vi "LVClass_SlopesPostProcessList AddProcessorTabWithVaraint.vi"(0 "SlopesPostProcessorList in":refnum<class "SlopesPostProcessorList.lvclass">, 7 "Processing list in":T1[](array[typedef]), 9 "Enum":enum16{"As new list", "Append", "InsertFront"}(ring), 11 "error in":errorcluster) -> (4 "SlopesPostProcessorList out":refnum<class "SlopesPostProcessorList.lvclass">, 15 "error out":errorcluster)   [LabVIEW 2020, in "SlopesPostProcessorList.lvclass"]
uses:
  SlopesPostProcessorList.lvclass
  SlopesPostProcessorList - ONE - with variant.ctl
  SlopesStructToVariant.ctl
  Point2D.ctl
  Point2Df.ctl
  Slopes origin - SlopesPostProcessingList.ctl
  HasoSlopes.lvclass
  PupillStructToVariant.ctl
  General dimensions definition.ctl
  Pupil.lvclass
  SlopesPostProcessorList - Double passage.ctl
  SlopesPostProcessorList - Filter.ctl
  SlopesPostProcessorList - Modulator.ctl
  SlopesPostProcessorList - Add lens.ctl
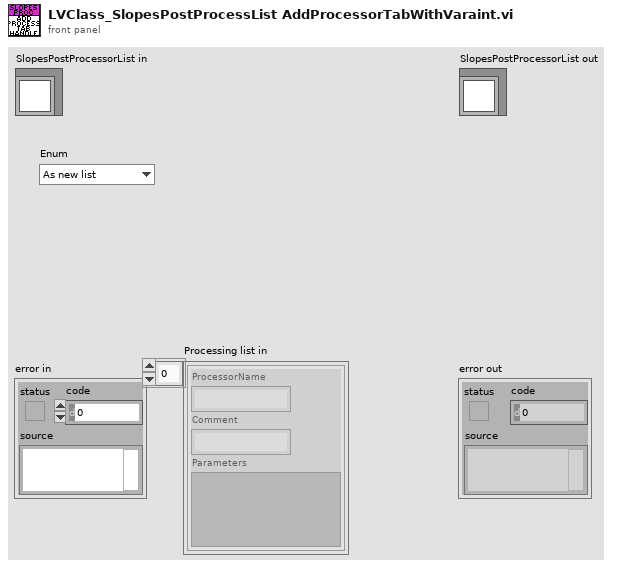
[diagram p1: front panel]
types:
  T1 = typedef "SlopesPostProcessorList - ONE - with variant.ctl" = cluster{"ProcessorName":string, "Comment":string, "Parameters":variant}
  T2 = typedef "SlopesPostProcessorList - Double passage.ctl" = cluster{"ActivateOnTilt":bool, "ActivateOnCurvature":bool}
  T3 = typedef "SlopesPostProcessorList - Filter.ctl" = cluster{"tiltx":bool, "tilty":bool, "curv":bool, "astig0":bool, "astig45":bool, "others":bool}
  T4 = typedef "SlopesPostProcessorList - Modulator.ctl" = cluster{"tiltx":sgl, "tilty":sgl, "curv":sgl, "astig0":sgl, "astig45":sgl, "others":sgl}
  T5 = typedef "SlopesPostProcessorList - Add lens.ctl" = cluster{"lens_m":sgl, "KeepCurvature":bool}
  T6 = typedef "SlopesStructToVariant.ctl" = cluster{"dimension":cluster{"size":T7, "step":T8}, "HASO serial number":string, "REF Type":T9, "Slopes from XML string format":string}
  T7 = typedef "Point2D.ctl" = cluster{"X":u32, "Y":u32}
  T8 = typedef "Point2Df.ctl" = cluster{"X":sgl, "Y":sgl}
  T9 = typedef "Slopes origin - SlopesPostProcessingList.ctl" = enum16{"Slopes from acq", "Slopes from file", "Slopes from data"}
  T10 = typedef "PupillStructToVariant.ctl" = cluster{"Dimension":T11, "Data":i32[][]}
  T11 = typedef "General dimensions definition.ctl" = cluster{"Size":T7, "Step":T8}
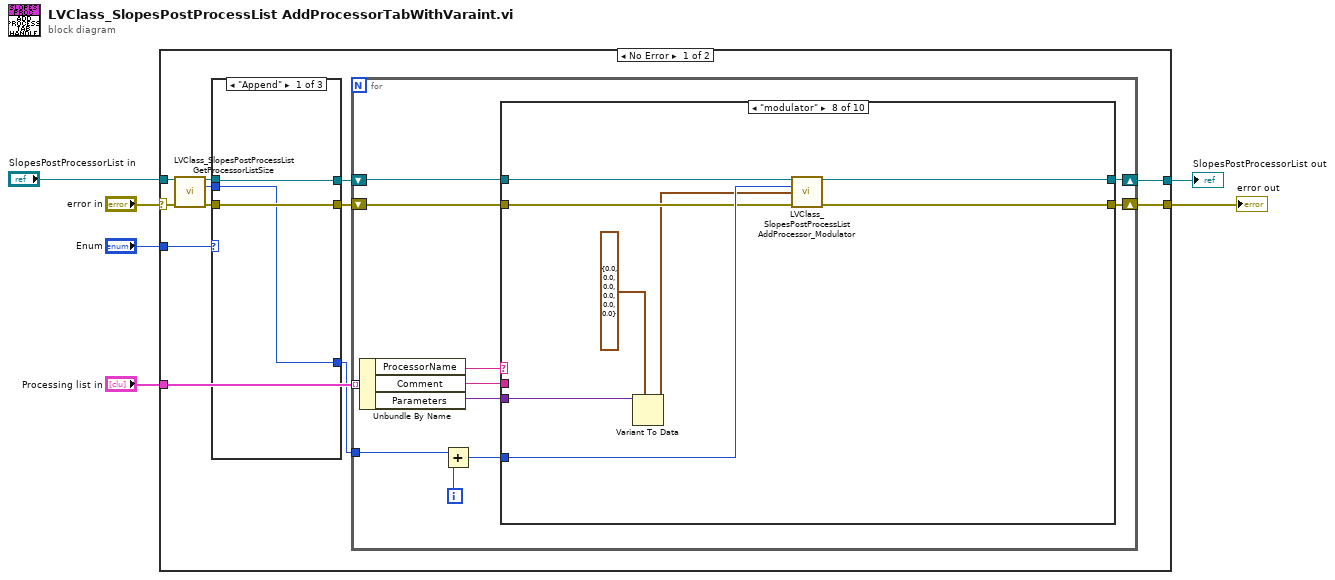
[diagram p0: block diagram]
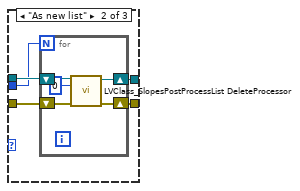
[diagram p2: hidden frame]
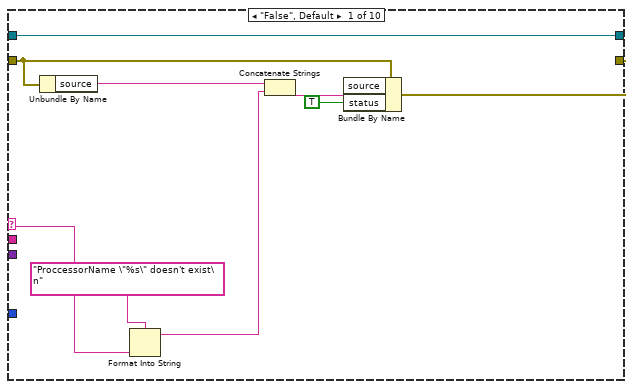
[diagram p4: hidden frame]
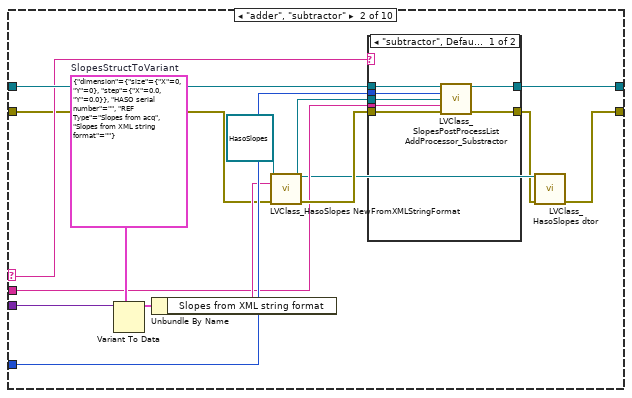
[diagram p5: hidden frame]
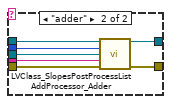
[diagram p6: hidden frame]
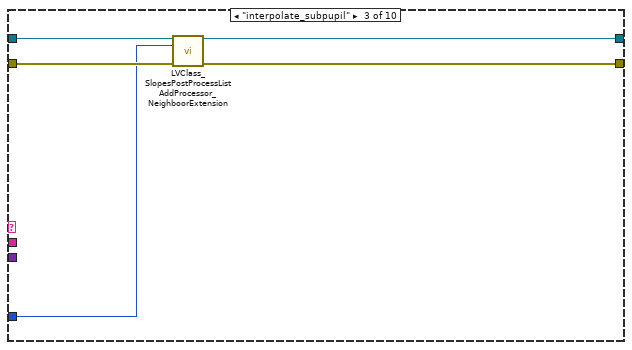
[diagram p7: hidden frame]
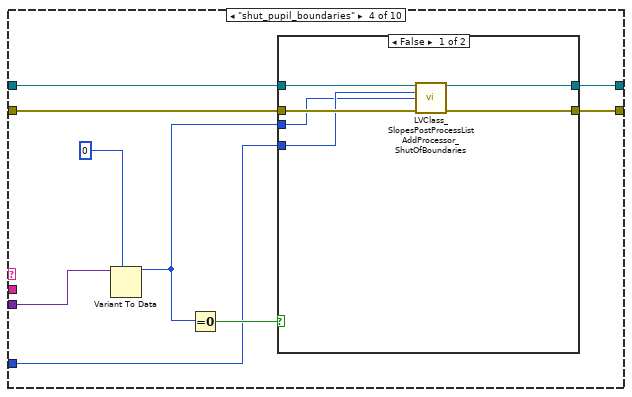
[diagram p8: hidden frame]
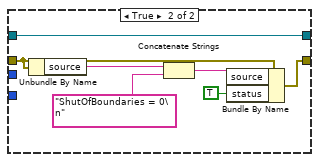
[diagram p9: hidden frame]
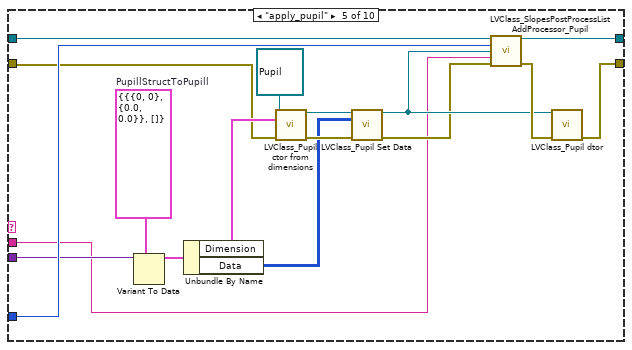
[diagram p10: hidden frame]
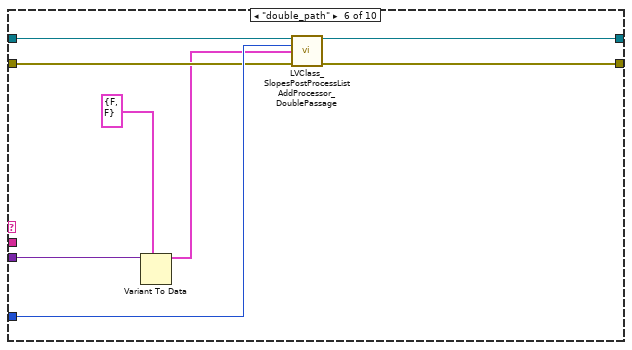
[diagram p11: hidden frame]
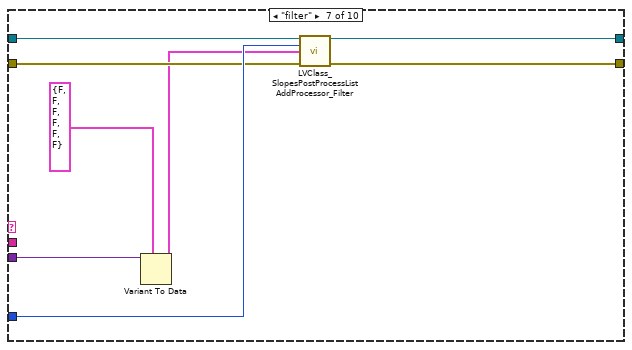
[diagram p12: hidden frame]
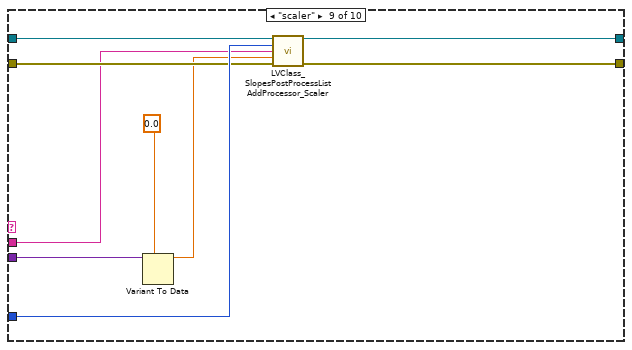
[diagram p13: hidden frame]
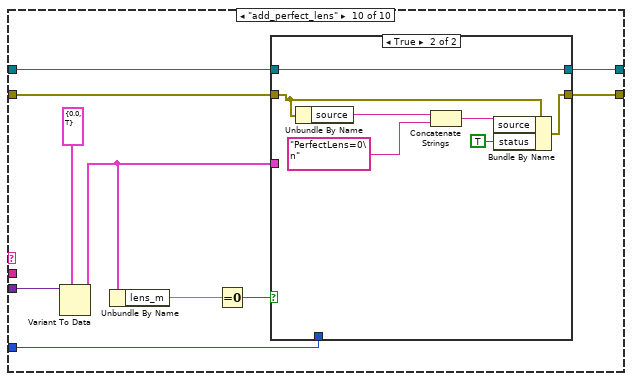
[diagram p14: hidden frame]
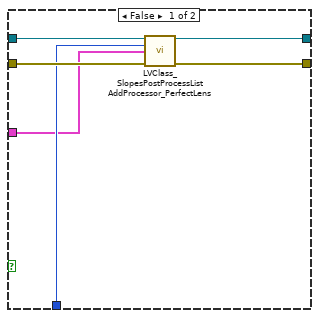
[diagram p15: hidden frame]
diagram:
  n1 = case shown="No Error" "error in" {
    selector: "error in" -> [w15 w184]
    tunnel: [w16 w184] -> w5
    tunnel: [w17 w183] -> w6
    tunnel: "SlopesPostProcessorList in" -> [w14 w183]
    tunnel: "Processing list in" -> [w18 _]
    tunnel: "Enum" -> [w9 _]
    frame No Error {
      n2 = call "LVClass_SlopesPostProcessList GetProcessorListSize.vi"("SlopesPostProcessorList in"=w14, "error in (no error)"=w15) -> ("SlopesPostProcessorList out"=w13:refnum<class "SlopesPostProcessorList.lvclass">, "size"=w8:u32, "error out"=w11:errorcluster)  [unwired: 11 in]
      n3 = case shown="\"Append\"" w9 {
        tunnel: w13 -> [w21 w26 w33]
        tunnel: [w21 w25 w33] -> w12
        tunnel: w11 -> [w20 w24 w32]
        tunnel: [w20 w23 w32] -> w10
        tunnel: w8 -> [w19 w22 _]
        tunnel: [w19 _ _] -> w7
        frame "Append" {
        }
        frame "As new list" {
          n4 = for {
            N: w22 -> [_]
            shift-right: [w30] -> w25
            shift-left: w26 -> [w31]
            shift-right: [w28] -> w23
            shift-left: w24 -> [w29]
            n5 = call "LVClass_SlopesPostProcessList DeleteProcessor.vi"("SlopesPostProcessorList in"=w31, "Position"=0, "error in (no error)"=w29) -> ("SlopesPostProcessorList out"=w30:refnum<class "SlopesPostProcessorList.lvclass">, "error out"=w28:errorcluster)  [unwired: 11 in]
          }
        }
        frame "InsertFront" {
        }
      }
      n6 = for {
        tunnel: w18 -> [w35] mode=indexing
        shift-right: [w42] -> w16
        shift-left: w10 -> [w43]
        shift-right: [w40] -> w17
        shift-left: w12 -> [w41]
        tunnel: w7 -> [w37]
        i -> [w39]
        n7 = Unbundle By Name(w35) -> ("ProcessorName"=w44:string, "Comment"=w34:string, "Parameters"=w36:variant)
        n8 = Add(x=w37, y=w39) -> (x+y=w38:u32)
        n9 = case shown="\"modulator\"" w44 {
          selector: w44 -> [w45 w65 _ _ _ _ _ _ _ _]
          tunnel: w43 -> [w53 w59 w85 w95 w113 w131 w139 w147 w156 w168]
          tunnel: [w52 w54 w84 w94 w120 w130 w137 w145 w155 w169] -> w42
          tunnel: w38 -> [_ w66 w83 w91 w125 w134 w141 w149 w157 w164]
          tunnel: w41 -> [w46 w68 w87 w93 w124 w133 w140 w148 w159 w166]
          tunnel: [w46 w67 w86 w92 w126 w132 w138 w146 w158 w165] -> w40
          tunnel: w36 -> [_ w63 _ w88 w122 w128 w142 w150 w152 w163]
          tunnel: w34 -> [_ w57 _ _ w110 _ _ _ w154 _]
          frame "False", Default {
            n10 = Unbundle By Name(w53) -> ("source"=w50:string)
            n11 = Format Into String(format string="ProccessorName \"%s\" doesn't exist\n" ("source"), w45) -> (resulting string=w48:string)  [unwired: 2 in, 1 out]
            n12 = Concatenate Strings(w50, w48) -> (w49:string)
            n13 = Bundle By Name(cluster=w53, "source"=w49, "status"=TRUE) -> (w52:errorcluster)
          }
          frame "adder", "subtractor" {
            w64 = T6 {"dimension"={"size"={"X"=0, "Y"=0}, "step"={"X"=0.0, "Y"=0.0}}, "HASO serial number"="", "REF Type"=enum."Slopes from acq", "Slopes from XML string format"=""}  # SlopesStructToVariant
            n14 = Variant To Data(type=w64, Variant=w63) -> (data=w62:T6)  [unwired: 1 in, 1 out]
            n15 = Unbundle By Name(w62) -> ("Slopes from XML string format"=w61:string)
            n16 = call "LVClass_HasoSlopes NewFromXMLStringFormat.vi"("HasoSlopes in"=refnum<class "HasoSlopes.lvclass"> refnum, "XML txt format"=w61, "error in (no error)"=w59) -> ("HasoSlopes out"=w56:refnum<class "HasoSlopes.lvclass">, "error out"=w58:errorcluster)  [unwired: 11 in]
            n17 = case shown="\"subtractor\", Default" w65 {
              tunnel: w68 -> [w75 w82]
              tunnel: [w70 w81] -> w67
              tunnel: w66 -> [w74 w80]
              tunnel: w57 -> [w72 w79]
              tunnel: w56 -> [w73 w78]
              tunnel: w58 -> [w71 w77]
              tunnel: [w69 w76] -> w55
              frame "subtractor", Default {
                n18 = call "LVClass_SlopesPostProcessList AddProcessor_Substractor.vi"("SlopesPostProcessorList in"=w75, "Position"=w74, "HasoSlopes.lvclass"=w73, "Comment"=w72, "error in (no error)"=w71) -> ("SlopesPostProcessorList out"=w70:refnum<class "SlopesPostProcessorList.lvclass">, "error out"=w69:errorcluster)  [unwired: 9 in]
              }
              frame "adder" {
                n19 = call "LVClass_SlopesPostProcessList AddProcessor_Adder.vi"("SlopesPostProcessorList in"=w82, "Position"=w80, "HasoSlopes.lvclass"=w78, "Comment"=w79, "error in (no error)"=w77) -> ("SlopesPostProcessorList out"=w81:refnum<class "SlopesPostProcessorList.lvclass">, "error out"=w76:errorcluster)  [unwired: 9 in]
              }
            }
            n20 = call "LVClass_HasoSlopes dtor.vi"("HasoSlopes in"=w56, "error in (no error)"=w55) -> ("error out"=w54:errorcluster)  [unwired: 12 in, 1 out]
          }
          frame "interpolate_subpupil" {
            n21 = call "LVClass_SlopesPostProcessList AddProcessor_NeighboorExtension.vi"("SlopesPostProcessorList in"=w87, "Position"=w83, "error in (no error)"=w85) -> ("SlopesPostProcessorList out"=w86:refnum<class "SlopesPostProcessorList.lvclass">, "error out"=w84:errorcluster)  [unwired: 11 in]
          }
          frame "shut_pupil_boundaries" {
            n22 = Variant To Data(type=u32 0 ("ShutOfBoundaries"), Variant=w88) -> (data=w89:u32)  [unwired: 1 in, 1 out]
            n23 = Equal To 0?(x=w89) -> (x = 0?=w96:bool)
            n24 = case shown="False" w96 {
              tunnel: w95 -> [w101 w104]
              tunnel: [w100 w105] -> w94
              tunnel: w93 -> [w102 w103]
              tunnel: [w99 w103] -> w92
              tunnel: w91 -> [w98 _]
              tunnel: w89 -> [w97 _]
              frame False {
                n25 = call "LVClass_SlopesPostProcessList AddProcessor_ShutOfBoundaries.vi"("SlopesPostProcessorList in"=w102, "Position"=w98, "ShutOfBoundaries"=w97, "error in (no error)"=w101) -> ("SlopesPostProcessorList out"=w99:refnum<class "SlopesPostProcessorList.lvclass">, "error out"=w100:errorcluster)  [unwired: 10 in]
              }
              frame True {
                n26 = Unbundle By Name(w104) -> ("source"=w108:string)
                n27 = Concatenate Strings(w108, "ShutOfBoundaries = 0\n" ("source")) -> (w107:string)
                n28 = Bundle By Name(cluster=w104, "source"=w107, "status"=TRUE) -> (w105:errorcluster)
              }
            }
          }
          frame "apply_pupil" {
            w123 = T10 {"Dimension"={"Size"={"X"=0, "Y"=0}, "Step"={"X"=0.0, "Y"=0.0}}, "Data"=[]}  # PupillStructToPupill
            n29 = Variant To Data(type=w123, Variant=w122) -> (data=w115:T10)  [unwired: 1 in, 1 out]
            n30 = Unbundle By Name(w115) -> ("Dimension"=w114:T11, "Data"=w111:i32[][])
            n31 = call "LVClass_Pupil ctor from dimensions.vi"("Pupil in"=refnum<class "Pupil.lvclass"> refnum, "Dimensions_um"=w114, "error in (no error)"=w113) -> ("Pupil out"=w116:refnum<class "Pupil.lvclass">, "error out"=w117:errorcluster)  [unwired: 11 in]
            n32 = call "LVClass_Pupil Set Data.vi"("Pupil in"=w116, "Data"=w111, "error in (no error)"=w117) -> ("Pupil out"=w119:refnum<class "Pupil.lvclass">, "error out"=w118:errorcluster)  [unwired: 11 in]
            n33 = call "LVClass_SlopesPostProcessList AddProcessor_Pupil.vi"("SlopesPostProcessorList in"=w124, "Position"=w125, "Pupil.lvclass"=w119, "Comment"=w110, "error in (no error)"=w118) -> ("SlopesPostProcessorList out"=w126:refnum<class "SlopesPostProcessorList.lvclass">, "error out"=w121:errorcluster)  [unwired: 9 in]
            n34 = call "LVClass_Pupil dtor.vi"("Pupil in"=w119, "error in (no error)"=w121) -> ("error out"=w120:errorcluster)  [unwired: 12 in, 1 out]
          }
          frame "double_path" {
            n35 = Variant To Data(type=T2 {"ActivateOnTilt"=FALSE, "ActivateOnCurvature"=FALSE} ("doublePassage"), Variant=w128) -> (data=w127:T2)  [unwired: 1 in, 1 out]
            n36 = call "LVClass_SlopesPostProcessList AddProcessor_DoublePassage.vi"("SlopesPostProcessorList in"=w133, "Position"=w134, "doublePath"=w127, "error in (no error)"=w131) -> ("SlopesPostProcessorList out"=w132:refnum<class "SlopesPostProcessorList.lvclass">, "error out"=w130:errorcluster)  [unwired: 10 in]
          }
          frame "filter" {
            n37 = Variant To Data(type=T3 {"tiltx"=FALSE, "tilty"=FALSE, "curv"=FALSE, "astig0"=FALSE, "astig45"=FALSE, "others"=FALSE} ("Filter"), Variant=w142) -> (data=w135:T3)  [unwired: 1 in, 1 out]
            n38 = call "LVClass_SlopesPostProcessList AddProcessor_Filter.vi"("SlopesPostProcessorList in"=w140, "Position"=w141, "Filter"=w135, "error in (no error)"=w139) -> ("SlopesPostProcessorList out"=w138:refnum<class "SlopesPostProcessorList.lvclass">, "error out"=w137:errorcluster)  [unwired: 10 in]
          }
          frame "modulator" {
            n39 = Variant To Data(type=T4 {"tiltx"=0.0, "tilty"=0.0, "curv"=0.0, "astig0"=0.0, "astig45"=0.0, "others"=0.0} ("Modulator"), Variant=w150) -> (data=w143:T4)  [unwired: 1 in, 1 out]
            n40 = call "LVClass_SlopesPostProcessList AddProcessor_Modulator.vi"("SlopesPostProcessorList in"=w148, "Position"=w149, "Modulator"=w143, "error in (no error)"=w147) -> ("SlopesPostProcessorList out"=w146:refnum<class "SlopesPostProcessorList.lvclass">, "error out"=w145:errorcluster)  [unwired: 10 in]
          }
          frame "scaler" {
            n41 = Variant To Data(type=sgl 0.0 ("scaler"), Variant=w152) -> (data=w151:sgl)  [unwired: 1 in, 1 out]
            n42 = call "LVClass_SlopesPostProcessList AddProcessor_Scaler.vi"("SlopesPostProcessorList in"=w159, "Position"=w157, "comment"=w154, "scaler"=w151, "error in (no error)"=w156) -> ("SlopesPostProcessorList out"=w158:refnum<class "SlopesPostProcessorList.lvclass">, "error out"=w155:errorcluster)  [unwired: 9 in]
          }
          frame "add_perfect_lens" {
            n43 = Variant To Data(type=T5 {"lens_m"=0.0, "KeepCurvature"=TRUE} ("Perfect lens"), Variant=w163) -> (data=w161:T5)  [unwired: 1 in, 1 out]
            n44 = Unbundle By Name(w161) -> ("lens_m"=w167:sgl)
            n45 = Equal To 0?(x=w167) -> (x = 0?=w160:bool)
            n46 = case shown="True" w160 {
              tunnel: w168 -> [w172 w179]
              tunnel: [w173 w178] -> w169
              tunnel: w166 -> [w175 w176]
              tunnel: [w174 w176] -> w165
              tunnel: w164 -> [w171 _]
              tunnel: w161 -> [w170 _]
              frame False {
                n47 = call "LVClass_SlopesPostProcessList AddProcessor_PerfectLens.vi"("SlopesPostProcessorList in"=w175, "Position"=w171, "Perfect lens"=w170, "error in (no error)"=w172) -> ("SlopesPostProcessorList out"=w174:refnum<class "SlopesPostProcessorList.lvclass">, "error out"=w173:errorcluster)  [unwired: 10 in]
              }
              frame True {
                n48 = Unbundle By Name(w179) -> ("source"=w181:string)
                n49 = Concatenate Strings(w181, "PerfectLens=0\n" ("source")) -> (w180:string)
                n50 = Bundle By Name(cluster=w179, "source"=w180, "status"=TRUE) -> (w178:errorcluster)
              }
            }
          }
        }
      }
    }
    frame Error {
    }
  }
  "error out" <- w5
  "SlopesPostProcessorList out" <- w6
